vi "Publish Data.vi"(6 "Publish Time (Use Current Time)":timestamp, 8 "error in (no error)":errorcluster, 9 "Data to Publish":variant, 10 "Datum Name":string, 11 "IModel in":refnum<class "IModel.lvclass">) -> (0 "error out":errorcluster, 3 "IModel out":refnum<class "IModel.lvclass">)   [LabVIEW 2020, in "MVA Framework.lvlib" / "IModel.lvlib" / "IModel.lvclass"]
doc: "将数据（值）发布到中介总线。任何有权访问中介总线的参与者都可以观察到已发布的数据。"
uses:
  IModel.lvclass
  IObserver/IObserver/IObserver.lvclass/IObserver.ctl
  IModel.lvclass/IModel.ctl
  IMediator/PublishRequest/PublishRequest.lvclass
  IMediator/PublishRequest/PublishRequest.lvclass/PublishRequest.ctl
  IMediator/IMediator Messages/Publish Msg/Publish Msg.lvclass/Publish Msg.ctl
  composed-af-messages/Source/RoundTripMessage/RoundTripMessage.lvclass/RoundTripMessage.ctl
  <vilib>/ActorFramework/Message Enqueuer/Message Enqueuer.lvclass/Message Enqueuer.ctl
  composed-af-messages/Source/RoundTripMessage/Return Round-Trip Message.vi
  <vilib>/ActorFramework/Message Enqueuer/Enqueue.vi
  IMediator/IMediator Messages/Publish Msg/Publish Msg.lvclass
  composed-af-messages/Source/RoundTripMessage/RoundTripMessage.lvclass
  C:/Program Files/National Instruments/LabVIEW 2020/vi.lib/ActorFramework/Message/Message.lvclass
  <vilib>/Utility/error.llb/Error Cluster From Error Code.vi
  <vilib>/ActorFramework/Message Priority Queue/Priority Enqueue.vi
  IObserver/IObserver/IObserver.lvclass
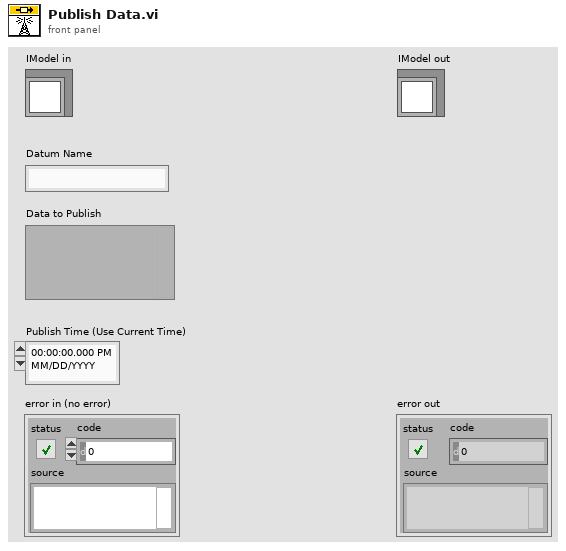
[diagram p1: front panel]
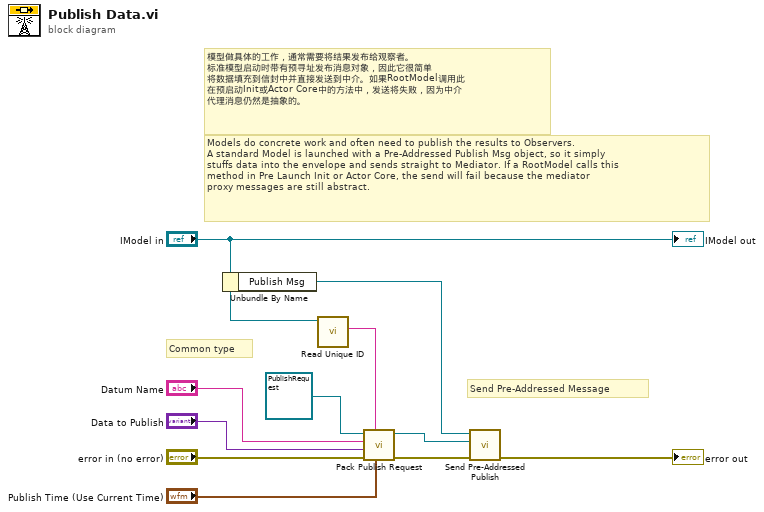
[diagram p0: block diagram]
diagram:
  # "模型做具体的工作，通常需要将结果发布给观察者。\n标准模型启动时带有预寻址发布消息对象，因此它很简单\n将数据填充到信封中并直接发送到中介。如果RootModel调用此\n在预启动Init或Actor Core中的方法中，发送将失败，因为中介\n代理消息仍然是抽象的。"
  # "Common type"
  # "Models do concrete work and often need to publish the results to Observers.\nA standard Model is launched with a Pre-Addressed Publish Msg object, so it simply\nstuffs data into the envelope and sends straight to Mediator. If a RootModel calls this\nmethod in Pre Launch Init or Actor Core, the send will fail because the mediator\nproxy messages are still abstract."
  # "Send Pre-Addressed Message"
  n1 = Unbundle By Name("IModel in") -> ("Publish Msg"=w11:refnum<class "Publish Msg.lvclass">)
  n2 = call "Read Unique ID.vi"("IObserver In"="IModel in") -> ("Unique ID"=w4:string)  [unwired: 10 in]
  n3 = call "Pack Publish Request.vi"("Publication Time (Use Current Time)"="Publish Time (Use Current Time)", "Publisher ID"=w4, "error in (no error)"="error in (no error)", "Value"="Data to Publish", "Datum Name"="Datum Name", "PublishRequest In"=refnum<class "PublishRequest.lvclass"> refnum ("IMediator.lvlib:PublishRequest.lvclass")) -> ("error out"=w2:errorcluster, "PublishRequest Out"=w5:refnum<class "PublishRequest.lvclass">)  [unwired: 4 in]
  n4 = call "Send Pre-Addressed Publish.vi"("error in (no error)"=w2, "PublishRequest"=w5, "Publish Message"=w11) -> ("error out"=→"error out":errorcluster)  [unwired: 8 in]
  "IModel out" <- "IModel in"
